vi "cases.vi"(9 "q 3":dbl(slide)=77.5 scale=0.0..200.0, 10 "q 2":dbl(slide)=85.0 scale=0.0..200.0, 11 "q 1":dbl(slide)=77.5 scale=0.0..200.0) -> (1 "q3":dbl, 2 "q2":dbl, 3 "q1":dbl)   [LabVIEW 2024]
panel:
  out "s? t:f":dbl[](array[numeric])
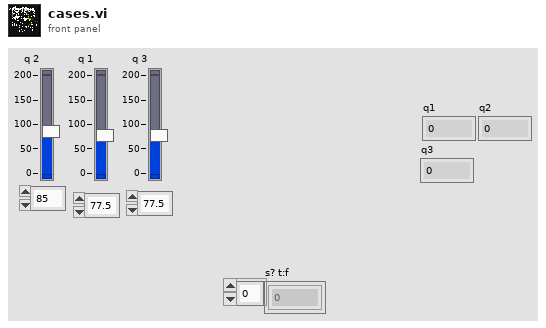
[diagram p1: front panel]
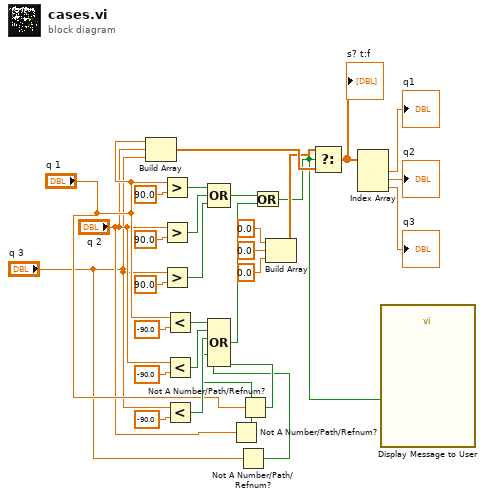
[diagram p0: block diagram]
diagram:
  n1 = Build Array("q 1", "q 2", "q 3") -> (w9:dbl[])
  n2 = Greater?(x="q 1", y=90.0) -> (0:w27:bool)
  n3 = Greater?(x="q 2", y=90.0) -> (0:w26:bool)
  n4 = Greater?(x="q 3", y=90.0) -> (0:w25:bool)
  n5 = Less?(x="q 1", y=-90.0) -> (x < y?=w21:bool)
  n6 = Less?(x="q 2", y=-90.0) -> (x < y?=w20:bool)
  n7 = Less?(x="q 3", y=-90.0) -> (x < y?=w19:bool)
  n8 = Compound Arithmetic op=OR(w27, w26, w25) -> (w18:bool)
  n9 = Not A Number/Path/Refnum?(number/path/refnum="q 2") -> (NaN/Path/Refnum?=w3:bool)
  n10 = Not A Number/Path/Refnum?(number/path/refnum="q 3") -> (NaN/Path/Refnum?=w2:bool)
  n11 = Not A Number/Path/Refnum?(number/path/refnum="q 1") -> (NaN/Path/Refnum?=w4:bool)
  n12 = Compound Arithmetic op=OR(w21, w20, w19, w4, w3, w2) -> (w17:bool)
  n13 = Or(x=w18, y=w17) -> (x .or. y?=w1:bool)
  n14 = Build Array(0.0 ("element"), 0.0 ("element"), 0.0 ("element")) -> (w8:dbl[])
  n15 = Select(t=w8, s=w1, f=w9) -> (s? t:f=w13:dbl[])
  "s? t:f" <- w13
  n16 = Index Array(array=w13) -> (element #1=→"q1":dbl, element #2=→"q2":dbl, element #3=→"q3":dbl)  [unwired: 3 in]
  n17 = call "Display Message to User"("Enable"=w1) -> ()  [unwired: 9 in, 2 out]
